vi "marshalling.vi"(8 "error in (no error)":errorcluster, 10 "Variant":variant, 11 "Serializer.Base64 in":refnum<class "Serializer.Base64.lvclass">) -> (0 "error out":errorcluster, 2 "String":string, 3 "Serializer.Base64 out":refnum<class "Serializer.Base64.lvclass">)   [LabVIEW 2013, in "Serializer.Base64.lvclass"]
uses:
  Serializer.Base64.lvclass
  <vilib>/Utility/GetType.llb/Type Enum.ctl
  Serializer.Base64.lvclass/Serializer.Base64.ctl
  <vilib>/LabVIEW Open Source Project/OpenSerializer/Serializer.FlattenedString/Serializer.FlattenedString.lvclass
  <vilib>/LabVIEW Open Source Project/Data Manipulation/TypeDescriptor/TypeDescriptor_GetType.vi
  <vilib>/Utility/GetType.llb/Get Type Code from I16 Array And Pos.vi
  <vilib>/LabVIEW Open Source Project/Data Manipulation/Variant/OpenVariant.lvlib
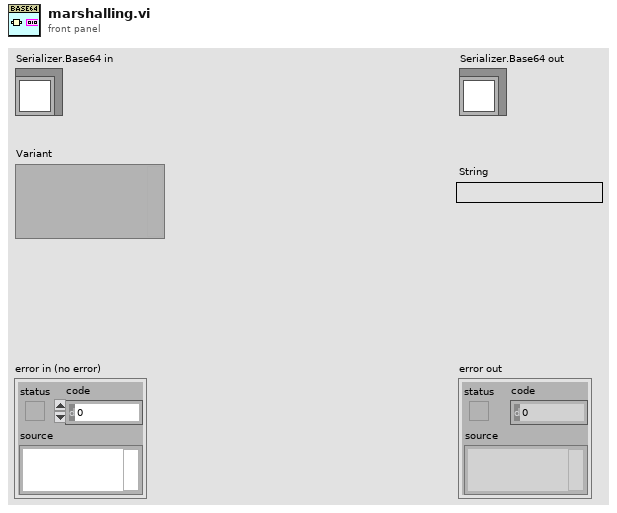
[diagram p1: front panel]
types:
  T1 = typedef "Type Enum.ctl" = enum8{"Void", "I8", "I16", "I32", "I64", "U8", "U16", "U32", "U64", "Single Float", "Double Float", "Extended Float", "Single Complex", "Double Complex", "Extended Complex", "Enum I8 NEVER", "Enum I16 NEVER", "Enum I32 NEVER", "Enum I64 NEVER", "Enum U8", "Enum U16", "Enum U32", "Enum U64", "Single Float With Unit", "Double Float With Unit", "Extended Float With Unit", "Single Complex With Unit", "Double Complex With Unit", "Extended Complex With Unit", "boolU16", "Boolean", "String", "Handle", "Path", "Picture", "C String", "Pascal String", "Tag", "SubString", "Array", "SubArray", "Cluster", "Numeric Cluster", "Variant", "LV Variant", "Measure Data (waveform)", "Refnum", "ExtData", "function", "Typedef", "Poly VI", "bad wire", "LabVIEW Class Instance"}
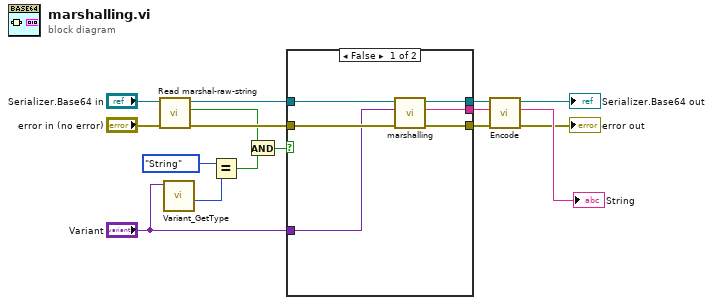
[diagram p0: block diagram]
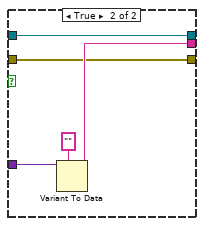
[diagram p2: hidden frame]
diagram:
  n1 = call "Read marshal-raw-string.vi"("error in (no error)"="error in (no error)", "Serializer.Base64 in"="Serializer.Base64 in") -> ("error out"=w7:errorcluster, "marshal-raw-string"=w2:bool, "Serializer.Base64 out"=w9:refnum<class "Serializer.Base64.lvclass">)  [unwired: 7 in]
  n2 = call <vilib>:"Variant_GetType.vi"("Variant"="Variant") -> ("Type Enum"=w5:T1)  [unwired: 8 in, 2 out]
  n3 = Equal?(x=Type_Enum."String", y=w5) -> (x = y?=w3:bool)
  n4 = And(x=w2, y=w3) -> (x .and. y?=w1:bool)
  n5 = case shown="False" w1 {
    tunnel: [w22 w25] -> w16
    tunnel: [w21 w23] -> w14
    tunnel: [w20 w24] -> w12
    tunnel: w9 -> [w19 w24]
    tunnel: w7 -> [w18 w23]
    tunnel: "Variant" -> [w17 w27]
    frame False {
      n6 = call-parent "marshalling.vi"("error in (no error)"=w18, "Variant"=w17, "Serializer in"=w19) -> ("error out"=w21:errorcluster, "String"=w22:string, "Serializer out"=w20:refnum<class "Serializer.Base64.lvclass">)  [unwired: 6 in]
    }
    frame True {
      n7 = Variant To Data(type="", Variant=w27) -> (data=w25:string)  [unwired: 1 in, 1 out]
    }
  }
  n8 = call "Encode.vi"("error in (no error)"=w14, "String"=w16, "Serializer.Base64 in"=w12) -> ("error out"=→"error out":errorcluster, "encoded string"=→"String":string, "Serializer.Base64 out"=→"Serializer.Base64 out":refnum<class "Serializer.Base64.lvclass">)  [unwired: 6 in]
